vi "SR830 set sensitivity.vi"(8 "error in (no error)":errorcluster, 10 "Sensitivity":T1 items=["2 nV", "5 nV", "10 nV", "20 nV", "50 nV", "100 nV", "200 nV", "500 nV", "1 uV", "2 uV", "5 uV", "10 uV", "20 uV", "50 uV", "100 uV", "200 uV", "500 uV", "1 mV", "2 mV", "5 mV", "10 mV", "20 mV", "50 mV", "100 mV", "200 mV", "500 mV", "1 V"], 11 "VISA resource name":refnum<visa-resource-name>) -> (0 "error out":errorcluster, 3 "VISA resource name out":refnum<visa-resource-name>)   [LabVIEW 2023, in "SR830.lvlib"]
doc: "Sets the current reference mode (internal or external) of the lock-in amplifier."
uses:
  SR830.lvlib
  Sensitivity_in_library.ctl
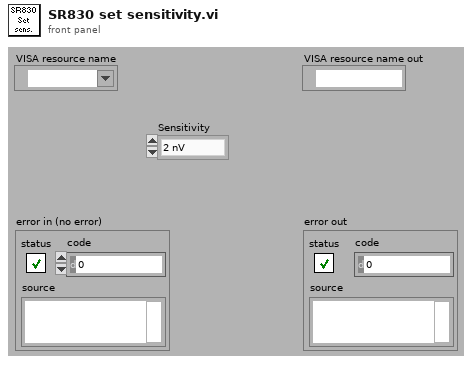
[diagram p1: front panel]
types:
  T1 = typedef "SR830.lvlib/Sensitivity_in_library.ctl" = u16
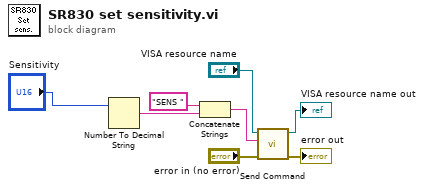
[diagram p0: block diagram]
diagram:
  n1 = Number To Decimal String(number="Sensitivity") -> (decimal integer string=w7:string)  [unwired: 1 in]
  n2 = Concatenate Strings("SENS " ("write buffer"), w7) -> (w6:string)
  n3 = call "Send Command.vi"("error in (no error)"="error in (no error)", "write buffer"=w6, "VISA resource name"="VISA resource name") -> ("error out"=→"error out":errorcluster, "VISA resource name out"=→"VISA resource name out":refnum<visa-resource-name>)  [unwired: 7 in]
